vi "Save Recall Instrument Status.vi"(8 "error in (no error)":errorcluster, 9 "Operation (0: Save)":i32(ring) items=["Save", "Recall"], 10 "Instrument State (0: State 0)":i32(ring) items=["State 0", "State 1", "State 2", "State 3", "State 4", "State 5", "State 6", "State 7", "State 8", "State 9"], 11 "VISA resource name":refnum<visa-resource-name>) -> (0 "error out":errorcluster, 3 "VISA resource name out":refnum<visa-resource-name>)   [LabVIEW 2020, in "Keysight E36300 Series.lvlib"]
doc: "Allows user to save current state to a non-volatile storage location or recall a previously stored state from one often non-volatile storage locations."
uses:
  Keysight E36300 Series.lvlib
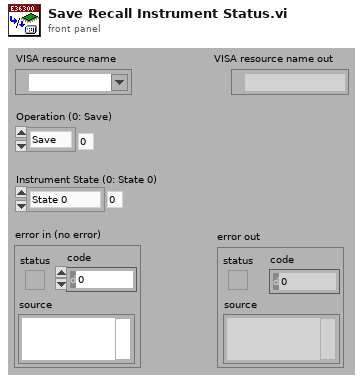
[diagram p1: front panel]
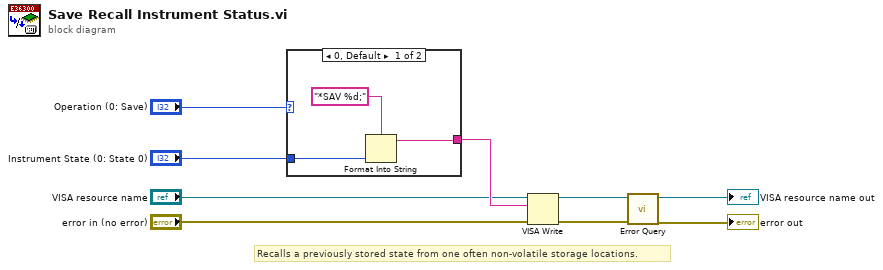
[diagram p0: block diagram]
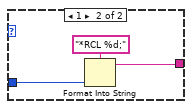
[diagram p2: hidden frame]
diagram:
  # "Recalls a previously stored state from one often non-volatile storage locations."
  n1 = case shown="0, Default" "Operation (0: Save)" {
    tunnel: "Instrument State (0: State 0)" -> [w12 w14]
    tunnel: [w11 w13] -> w8
    frame 0, Default {
      n2 = Format Into String(format string="*SAV %d;", w12) -> (resulting string=w11:string)  [unwired: 2 in, 1 out]
    }
    frame 1 {
      n3 = Format Into String(format string="*RCL %d;", w14) -> (resulting string=w13:string)  [unwired: 2 in, 1 out]
    }
  }
  n4 = VISA Write(VISA resource name="VISA resource name", write buffer=w8, error in (no error)="error in (no error)") -> (VISA resource name out=w5:refnum<visa-resource-name>, error out=w4:errorcluster)  [unwired: 1 out]
  n5 = call "Error Query.vi"("error in (no error)"=w4, "VISA resource name"=w5) -> ("error out"=→"error out":errorcluster, "VISA resource name out"=→"VISA resource name out":refnum<visa-resource-name>)  [unwired: 6 in, 2 out]
